vi "Time passed.vi"(1 "ms timer value":u32, 2 "Wait time":u32, 3 "Reset":bool) -> (0 "Boolean out":bool)   [LabVIEW 2019]
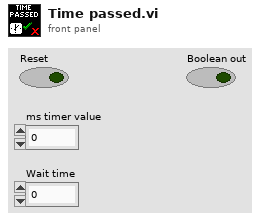
[diagram p1: front panel]
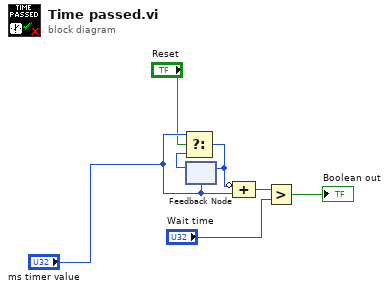
[diagram p0: block diagram]
diagram:
  n1 = feedback #1("ms timer value") -> (w1:u32)
  n2 = Select(t="ms timer value", s="Reset", f=w1) -> (s? t:f=w5:u32)
  n3 = feedback-in #1(w5) -> ()
  n4 = Compound Arithmetic op=ADD(invert w5, "ms timer value") -> (w6:u32)
  n5 = Greater?(x=w6, y="Wait time") -> (0:→"Boolean out":bool)
